vi "Test_Limiter.vi"() -> ()   [LabVIEW 2022 SP3]
panel:
  in  "LL":dbl
  out "BO1":bool
  out "AO1":dbl
  out "BO2":bool
  in  "AI3":dbl
  in  "AI2":dbl
  in  "AI1":dbl
  in  "UL":dbl
  in  "stop":bool
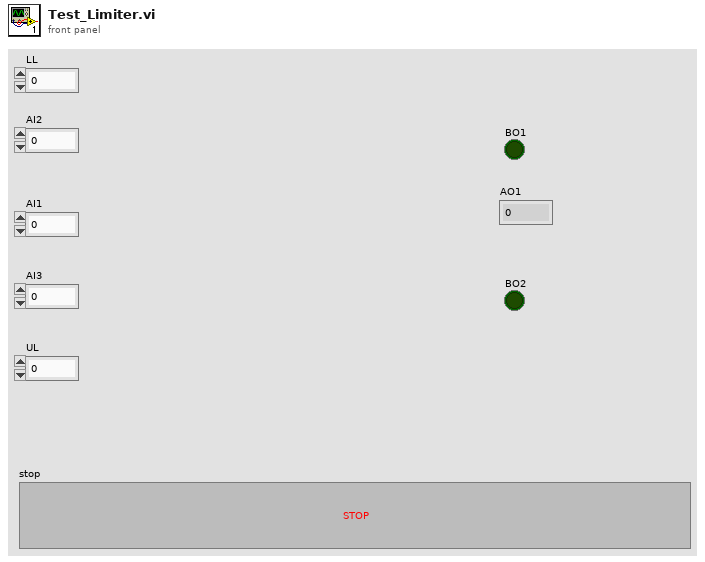
[diagram p1: front panel]
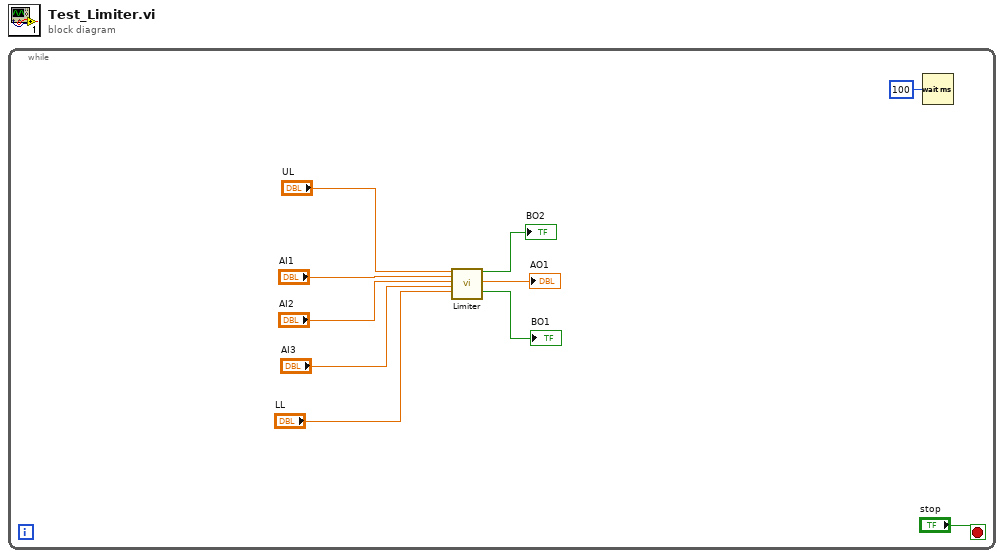
[diagram p0: block diagram]
diagram:
  n1 = while {
    stop <- "stop" stop-if-true
    n2 = call "Limiter.vi"("UL"="UL", "AI1"="AI1", "AI2"="AI2", "AI3"="AI3", "LL"="LL") -> ("BO2"=→"BO2":bool, "AO1"=→"AO1":dbl, "BO1"=→"BO1":bool)  [unwired: 11 in, 1 out]
    n3 = Wait (ms)(milliseconds to wait=u32 100) -> ()  [unwired: 1 out]
  }
